vi "Read Port.vi"(0 "Simulated Device in":refnum<class "Simulated Device.lvclass">, 5 "VISA resource name":refnum<visa-resource-name>, 7 "Port":dbl, 11 "error in (no error)":errorcluster) -> (4 "Simulated Device out":refnum<class "Simulated Device.lvclass">, 6 "VISA resource name 2":refnum<visa-resource-name>, 8 "Binary Number":T1, 10 "Response":string, 15 "error out":errorcluster)   [LabVIEW 2020, in "Simulated Device.lvclass"]
uses:
  Simulated Device.lvclass
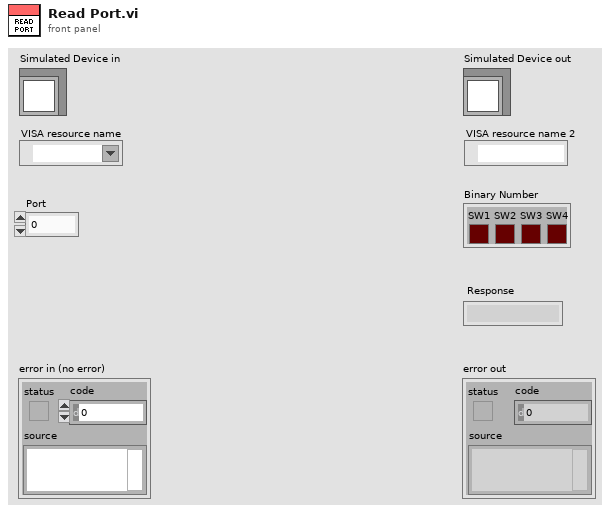
[diagram p1: front panel]
types:
  T1 = cluster{"SW1":bool, "SW2":bool, "SW3":bool, "SW4":bool, "[4]":bool, "[5]":bool, "[6]":bool, "[7]":bool, "[8]":bool}
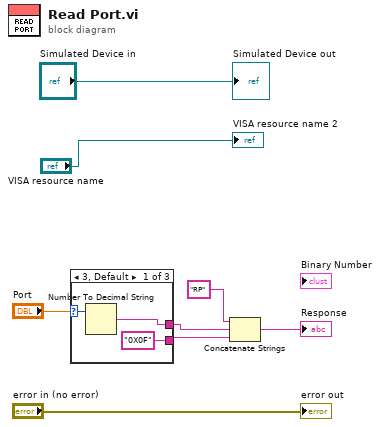
[diagram p0: block diagram]
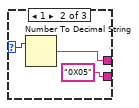
[diagram p2: hidden frame]
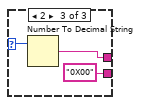
[diagram p3: hidden frame]
diagram:
  n1 = case shown="3, Default" "Port" {
    selector: "Port" -> [w11 w14 w17]
    tunnel: [w10 w13 w16] -> w3
    tunnel: ["0X0F" "0X05" "0X00"] -> w2
    frame 3, Default {
      n2 = Number To Decimal String(number=w11) -> (decimal integer string=w10:string)  [unwired: 1 in]
    }
    frame 1 {
      n3 = Number To Decimal String(number=w14) -> (decimal integer string=w13:string)  [unwired: 1 in]
    }
    frame 2 {
      n4 = Number To Decimal String(number=w17) -> (decimal integer string=w16:string)  [unwired: 1 in]
    }
  }
  n5 = Concatenate Strings("RP", w3, w2) -> (→"Response":string)
  "error out" <- "error in (no error)"
  "Simulated Device out" <- "Simulated Device in"
  "VISA resource name 2" <- "VISA resource name"
